vi "ideal direction.vi"(1 "Drone":T1) -> (0 "ideal direction":dbl(knob) scale=0.0..8.0)   [LabVIEW 2009]
uses:
  Drone data.ctl
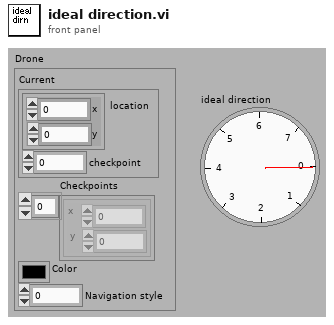
[diagram p1: front panel]
types:
  T1 = typedef "Drone data.ctl" = cluster{"Current":cluster{"location":cluster{"x":i16, "y":i16}, "checkpoint":i32}, "Checkpoints":cluster{"x":i16, "y":i16}[], "Color":u32, "Navigation style":i32}
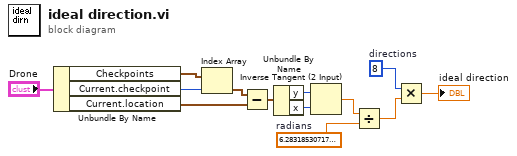
[diagram p0: block diagram]
diagram:
  w2 = 8  # directions
  w4 = 6.283185307179586  # radians
  n1 = Unbundle By Name("Drone") -> ("Checkpoints"=w12:cluster{"x":i16, "y":i16}[], "Current.checkpoint"=w11:i32, "Current.location"=w10:cluster{"x":i16, "y":i16})
  n2 = Index Array(array=w12, index=w11) -> (element=w9:cluster{"x":i16, "y":i16})
  n3 = Subtract(x=w9, y=w10) -> (x-y=w8:cluster{"x":i16, "y":i16})
  n4 = Unbundle By Name(w8) -> ("y"=w7:i16, "x"=w6:i16)
  n5 = Inverse Tangent (2 Input)(1:w6, 2:w7) -> (0:w5:dbl)
  n6 = Divide(x=w5, y=w4) -> (x/y=w3:dbl)
  n7 = Multiply(x=w2, y=w3) -> (x*y=→"ideal direction":dbl)
